vi "LIA_FPGA3a-PD Test-1.vi"() -> (1 "K Constant":fxp<+/-,32,16>, 2 "Nominal Freq":fxp<+/-,64,32>)   [LabVIEW 2012]
uses:
  <vilib>/rvi/DataTransferAndStorage/Container/Common/niFpgaContainerMetaDataKey.ctl
  <vilib>/rvi/DataTransferAndStorage/Container/Common/niFpgaContainerState.ctl
  <vilib>/rvi/DataTransferAndStorage/Container/Common/niFpgaDataTypeControl.ctl
  <vilib>/rvi/DataTransferAndStorage/Container/Common/niFpgaContainerImplementationControl.ctl
  <vilib>/rvi/DataTransferAndStorage/Container/Common/niFpgaContainerArbitrationOptionsControl.ctl
  <vilib>/rvi/DataTransferAndStorage/Container/Common/niFpgaTransferTypeControl.ctl
  <vilib>/rvi/DataTransferAndStorage/Container/Common/niFpgaContainerInitializationParameters.ctl
  <vilib>/rvi/Memory/Memory_Types/niFpgaMemoryInterfaceConfiguration.ctl
  <vilib>/rvi/FIFO/Fifo_Types/niFpgaFifoControlLogicControl.ctl
  <vilib>/Platform/TimedLoop/XDataNode/timing_clust.ctl
  <vilib>/Platform/TimedLoop/XDataNode/nitl_modes.ctl
  <vilib>/Platform/TimedLoop/XDataNode/wakeup.ctl
  <vilib>/rvi/FXPMathLib/FxpSinAndCos/subVIs/nifxpmath_SinAndCos_SimConfig.ctl
  <vilib>/rvi/FXPMathLib/basic elements/FxpIntAccumulator/subVIs/nifxpmath_IntAccumulator_SimConfig.ctl
  <vilib>/rvi/DataTransferAndStorage/Container/Common/niFpgaContainerGetUniqueNameForEmu.vi
  <vilib>/rvi/DataTransferAndStorage/Container/Common/niFpgaContainerSetEmuInfo.vi
  <vilib>/rvi/eio/common/nirviEmuReportErrorAndStop.vi
  <vilib>/rvi/FXPMathLib/FxpSinAndCos/simVIs/DllFxpSinAndCosTemp_sub.vi
  <vilib>/rvi/FXPMathLib/basic elements/FxpIntAccumulator/simVIs/DllFxpIntAccumulator_sub.vi
  <vilib>/rvi/eio/common/nirviEmuTemplateMethod_errors.vi
  <vilib>/rvi/Emulation/niFpgaSctlEmulationGetInTimedLoop.vi
  <vilib>/rvi/FIFO/Fifo_Resource/nirvififoEmulationSetSize.vi
  <vilib>/rvi/errors/niFpgaSetErrorForExecOnDevCompSimple.vi
  <vilib>/rvi/Emulation/niFpgaSctlEmulationFifoFullMgr.vi
  <vilib>/rvi/Emulation/niFpgaSctlEmulationResourceMgr.vi
  <vilib>/rvi/Emulation/niFpgaSctlEmulationRegisterWithScheduler.vi
  <vilib>/rvi/Emulation/niFpgaSctlEmulationScheduler.vi
  <vilib>/rvi/LocalResourceManager/LocalResourceManager.xnode
  <vilib>/Platform/TimedLoop/XDataNode/XDataNode.xnode
  <vilib>/rvi/FXPMathLib/FxpSinAndCos/XNode/nifxpmath_SinAndCos.xnode
  <vilib>/rvi/FXPMathLib/basic elements/FxpIntAccumulator/XNode/nifxpmath_IntAccumulator.xnode
  <vilib>/rvi/FXPMathLib/FxpInterpret/XNode/nifxpmath_Interpret.xnode
  <vilib>/eio/EIONode/EIONode.xnode
  <vilib>/rvi/DataTransferAndStorage/Container/XNode/niFpgaContainer.xnode
  <vilib>/rvi/FIFO/Fifo_Resource/nirvififoEmulationWrite.vi
  <vilib>/rvi/FIFO/Fifo_Resource/nirvififoEmulationRead.vi
  <vilib>/Platform/TimedLoop/XDataNode/XDNodeRunTimeDep.lvlib
panel:
  out "Sine Output":fxp<+/-,64,32>
  in  "Voltage (V)":fxp<+,64,12>=3276.8125
  in  "Z":fxp<+/-,64,16>
  out "Summation":fxp<+/-,64,32>
  out "Test Output":i16
  in  "Test":i16
  out "Radians":fxp<+/-,14,5>
  out "Cos":fxp<+/-,14,2>
  out "Sin":fxp<+/-,14,2>
  in  "Period":u16=1000
  out "ticks":u16
  out "ref":i16 format="%.0x"
  out "sig":i16 format="%.0x"
  out "channelQ":i64
  out "channelI":i64
  out "f":fxp<+/-,32,0> format="%.32g"
  in  "start":bool
  in  "dec2":i16=1
  in  "K":fxp<+,16,0>=0.001007080078125
  in  "nominal freq":fxp<+,16,0>=0.010009765625
  in  "dec1":i16=1
  in  "stages":i8=1
  in  "stop":bool
  in  "decimation":i16=1024
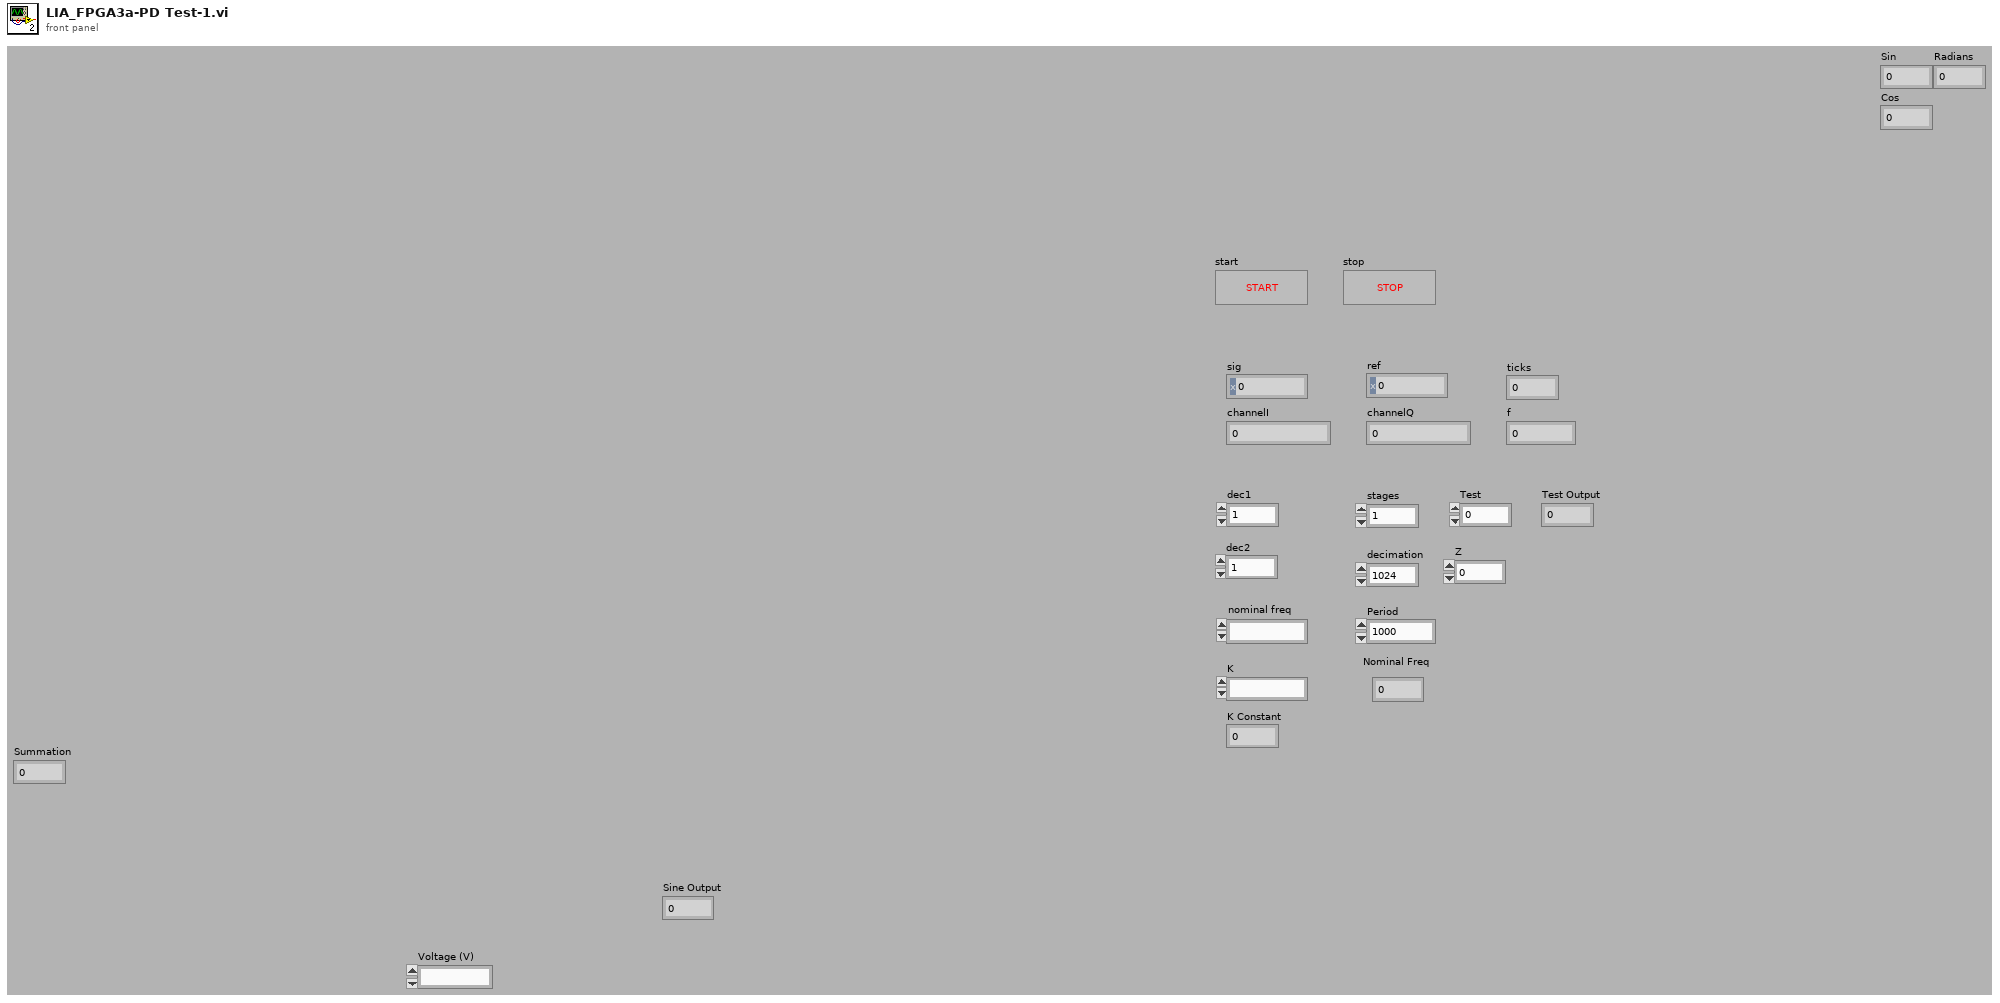
[diagram p1: front panel]
types:
  T1 = typedef "XDNodeRunTimeDep.lvlib/timing_clust.ctl" = cluster{"Expected End [f-1]":u64, "Actual End [f-1]":u64, "Finished Late? [f-1]":bool, "Expected End [i-1]":u64, "Actual End [i-1]":u64, "Finished Late? [i-1]":bool, "Expected Start [i]":u64, "Actual Start [i]":u64, "Expected Start [f]":u64, "Actual Start [f]":u64, "Source Name":string, "Structure Name":string, "Period":i64, "Deadline":i64, "Offset":i64, "Start":i64, "Priority":i32, "Timeout":i32, "Mode":T2, "Wakeup Reason":T3, "Error":errorcluster, "Source Type":string, "Secondary Source Type":string, "Global End Time":u64, "Global Start Time":u64, "Frame Duration":u64, "Iteration Duration":u64, "Assigned CPU":i32, "I/O Scan Engine Mode":u32}
  T2 = typedef "XDNodeRunTimeDep.lvlib/nitl_modes.ctl" = enum32{"No Change", "Process missed periods, maintain original phase", "Discard missed periods, maintain original phase", "Process missed periods, ignore original phase", "Discard missed periods, ignore original phase"}
  T3 = typedef "XDNodeRunTimeDep.lvlib/wakeup.ctl" = enum32{"Normal", "Aborted", "Asynchronous wakeup", "Timing source error", "Timed loop error", "Timeout"}
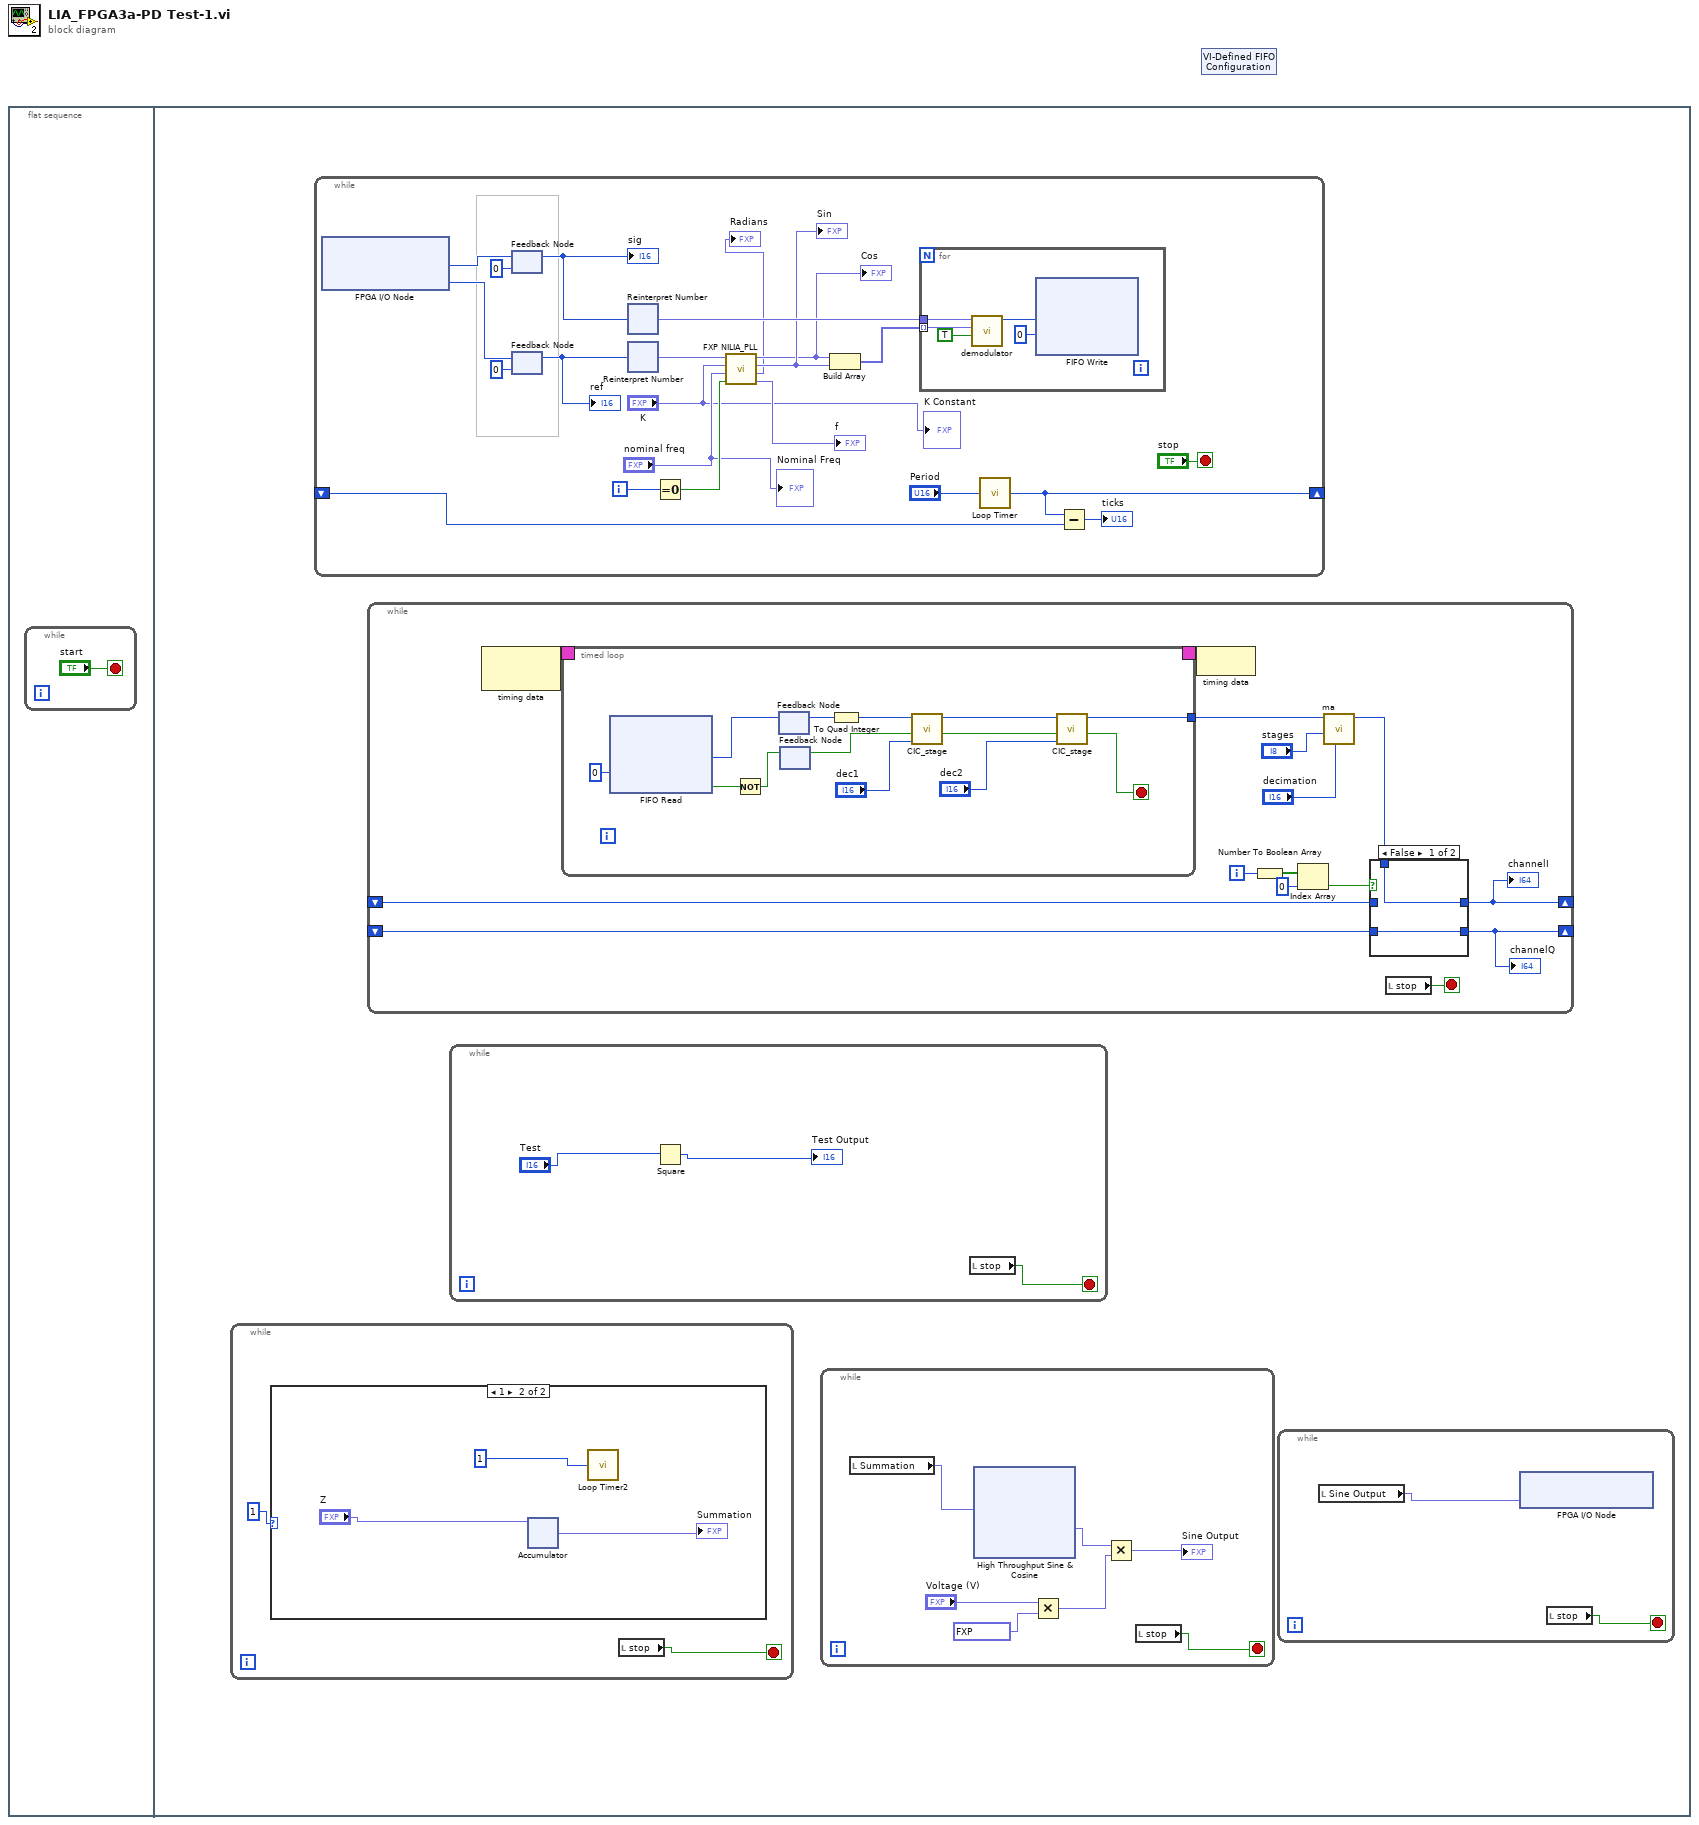
[diagram p0: block diagram]
diagram:
  n1 = flat-sequence {
    frame #0 {
      n2 = while {
        stop <- "start" stop-if-true
      }
    }
    frame #1 {
      n3 = while {
        stop <- w41 stop-if-true
        n4 = case shown="1" 1 {
          frame 0, Default {
          }
          frame 1 {
            n5 = xnode "Accumulator"("x"="Z") -> ("s"=→"Summation":fxp<+/-,64,16>)  [unwired: 4 in, 1 out]
            n6 = call "Loop Timer2"("Count(uSec)"=1) -> ()  [unwired: 1 out]
          }
        }
        n7 = local read "stop"() -> (w41:bool)
      }
      n8 = while {
        shift-right: [w94] -> _
        shift-left: _ -> [w93]
        i -> [w97]
        stop <- "stop" stop-if-true
        n9 = xnode "FPGA I/O Node"() -> ("Connector0/AI6"=w87:i16, "Connector0/AI7"=w84:i16)  [unwired: 2 in, 2 out]
        n10 = feedback #1(i16 0 ("y")) -> (w86:i16)
        "sig" <- w86
        n11 = feedback-in #1(w87) -> ()
        n12 = feedback #2(i16 0 ("z [I32.1]")) -> (w85:i16)
        "ref" <- w85
        n13 = feedback-in #2(w84) -> ()
        n14 = xnode "Reinterpret Number"("x"=w86) -> ("y"=w90:fxp<+/-,16,1>)
        n15 = xnode "Reinterpret Number"("x"=w85) -> ("y"=w83:fxp<+/-,16,1>)
        n16 = Equal To 0?(x=w97) -> (x = 0?=w81:bool)
        n17 = call "FXP NILIA_PLL.vi"("reset?"=w81, "norminal freq [U16.0]"="nominal freq", "alpha [U16.0]"="K", "x[I16.1]"=w83) -> ("f"=→"f":fxp<+/-,32,0>, "z [I32.1]"=→"Radians":fxp<+/-,32,1>, "sin(z)"=w78:fxp<+/-,16,2>, "cos(z)"=w77:fxp<+/-,16,2>)  [unwired: 4 in]
        "Sin" <- w78
        "Cos" <- w77
        n18 = Build Array(w77, w78) -> (w91:fxp<+/-,16,2>[])
        n19 = for {
          tunnel: w90 -> [w100]
          tunnel: w91 -> [w98] mode=indexing
          n20 = call "demodulator.vi"("New Data"=TRUE, "ref"=w98, "signal"=w100) -> ("x*y"=w101:i32)  [unwired: 8 out]
          n21 = xnode ("FIFO Write")("Element"=w101, "Timeout"=0) -> ()  [unwired: 1 in, 2 out]
        }
        n22 = call "Loop Timer"("Count(Ticks)"="Period") -> ("Tick Count(Ticks)"=w94:u16)
        n23 = Subtract(x=w94, y=w93) -> (x-y=→"ticks":u16)
        "Nominal Freq" <- "nominal freq"
        "K Constant" <- "K"
      }
      n24 = while {
        shift-right: [w104] -> _
        shift-left: _ -> [w106]
        shift-right: [w103] -> _
        shift-left: _ -> [w105]
        i -> [w111]
        stop <- w113 stop-if-true
        n25 = node-c288() -> (w117:T1)  [unwired: 1 out]
        n26 = timed-loop {
          timing: w117 -> [_]
          timing-out: [_] -> w116
          tunnel: [w125] -> w112
          stop <- w124 stop-if-true
          n27 = xnode ("FIFO Read")("Timeout"=0) -> ("Element"=w132:i32, "Timed Out?"=w131:bool)  [unwired: 1 in, 1 out]
          n28 = Not(x=w131) -> (.not. x?=w130:bool)
          n29 = feedback-in #3(w132) -> ()
          n30 = feedback #3() -> (w134:i32)  [unwired: 1 out]
          n31 = feedback-in #4(w130) -> ()
          n32 = feedback #4() -> (w128:bool)  [unwired: 1 out]
          n33 = To Quad Integer(1:w134) -> (0:w129:i64)
          n34 = call "CIC_stage.vi"("decimate factor"="dec1", "New Data"=w128, "input"=w129) -> ("Data Ready"=w126:bool, "output"=w127:i64)  [unwired: 7 out]
          n35 = call "CIC_stage.vi"("decimate factor"="dec2", "New Data"=w126, "input"=w127) -> ("Data Ready"=w124:bool, "output"=w125:i64)  [unwired: 7 out]
        }
        n36 = node-c288(w116) -> ()
        n37 = Number To Boolean Array(number=w111) -> (Boolean array=w110:bool[])
        n38 = Index Array "Index Array"(array=w110, index=0) -> (element=w108:bool)
        n39 = call "ma.vi"("decimate"="decimation", "stages"="stages", "input"=w112) -> ("output"=w107:i64)  [unwired: 8 out]
        n40 = case shown="False" w108 {
          tunnel: w107 -> [w119 w121]
          tunnel: [w119 w120] -> w104
          tunnel: [w118 w121] -> w103
          tunnel: w106 -> [_ w120]
          tunnel: w105 -> [w118 _]
          frame False {
          }
          frame True {
          }
        }
        "channelI" <- w104
        "channelQ" <- w103
        n41 = local read "stop"() -> (w113:bool)
      }
      n42 = while {
        stop <- w75 stop-if-true
        n43 = Square(x="Test") -> (x^2=→"Test Output":i16)
        n44 = local read "stop"() -> (w75:bool)
      }
      n45 = while {
        stop <- w4 stop-if-true
        n46 = local read "Summation"() -> (w10:fxp<+/-,64,32>)
        n47 = xnode "High Throughput Sine & Cosine"("x (pi)"=w10) -> ("sin(x)"=w9:fxp<+/-,16,2>)  [unwired: 1 out]
        n48 = Multiply(x="Voltage (V)", y=fxp<+,17,12> 3276.8125) -> (x*y=w5:fxp<+,64,24>)
        n49 = Multiply(x=w9, y=w5) -> (x*y=→"Sine Output":fxp<+/-,64,26>)
        n50 = local read "stop"() -> (w4:bool)
      }
      n51 = while {
        stop <- w2 stop-if-true
        n52 = local read "Sine Output"() -> (w3:fxp<+/-,64,32>)
        n53 = xnode "FPGA I/O Node"("Connector0/AO2"=w3) -> ()  [unwired: 1 in, 1 out]
        n54 = local read "stop"() -> (w2:bool)
      }
    }
  }
  n55 = xnode "VI-Defined FIFO Configuration"() -> ()  [unwired: 1 out]
